vi "KB_GetCreatFlatnessXYZ.vi"(10 "Recent":dbl[](array[numeric]), 11 "Image Pixels (U8)":dbl[][](array[numeric])) -> (3 "Create Flatnesss Base Point":cluster{"X":dbl, "Y":dbl, "Z":dbl}[](array[cluster]))   [LabVIEW 2015]
panel:
  out "输出簇":cluster{"X":dbl, "Y":dbl, "Z":dbl}
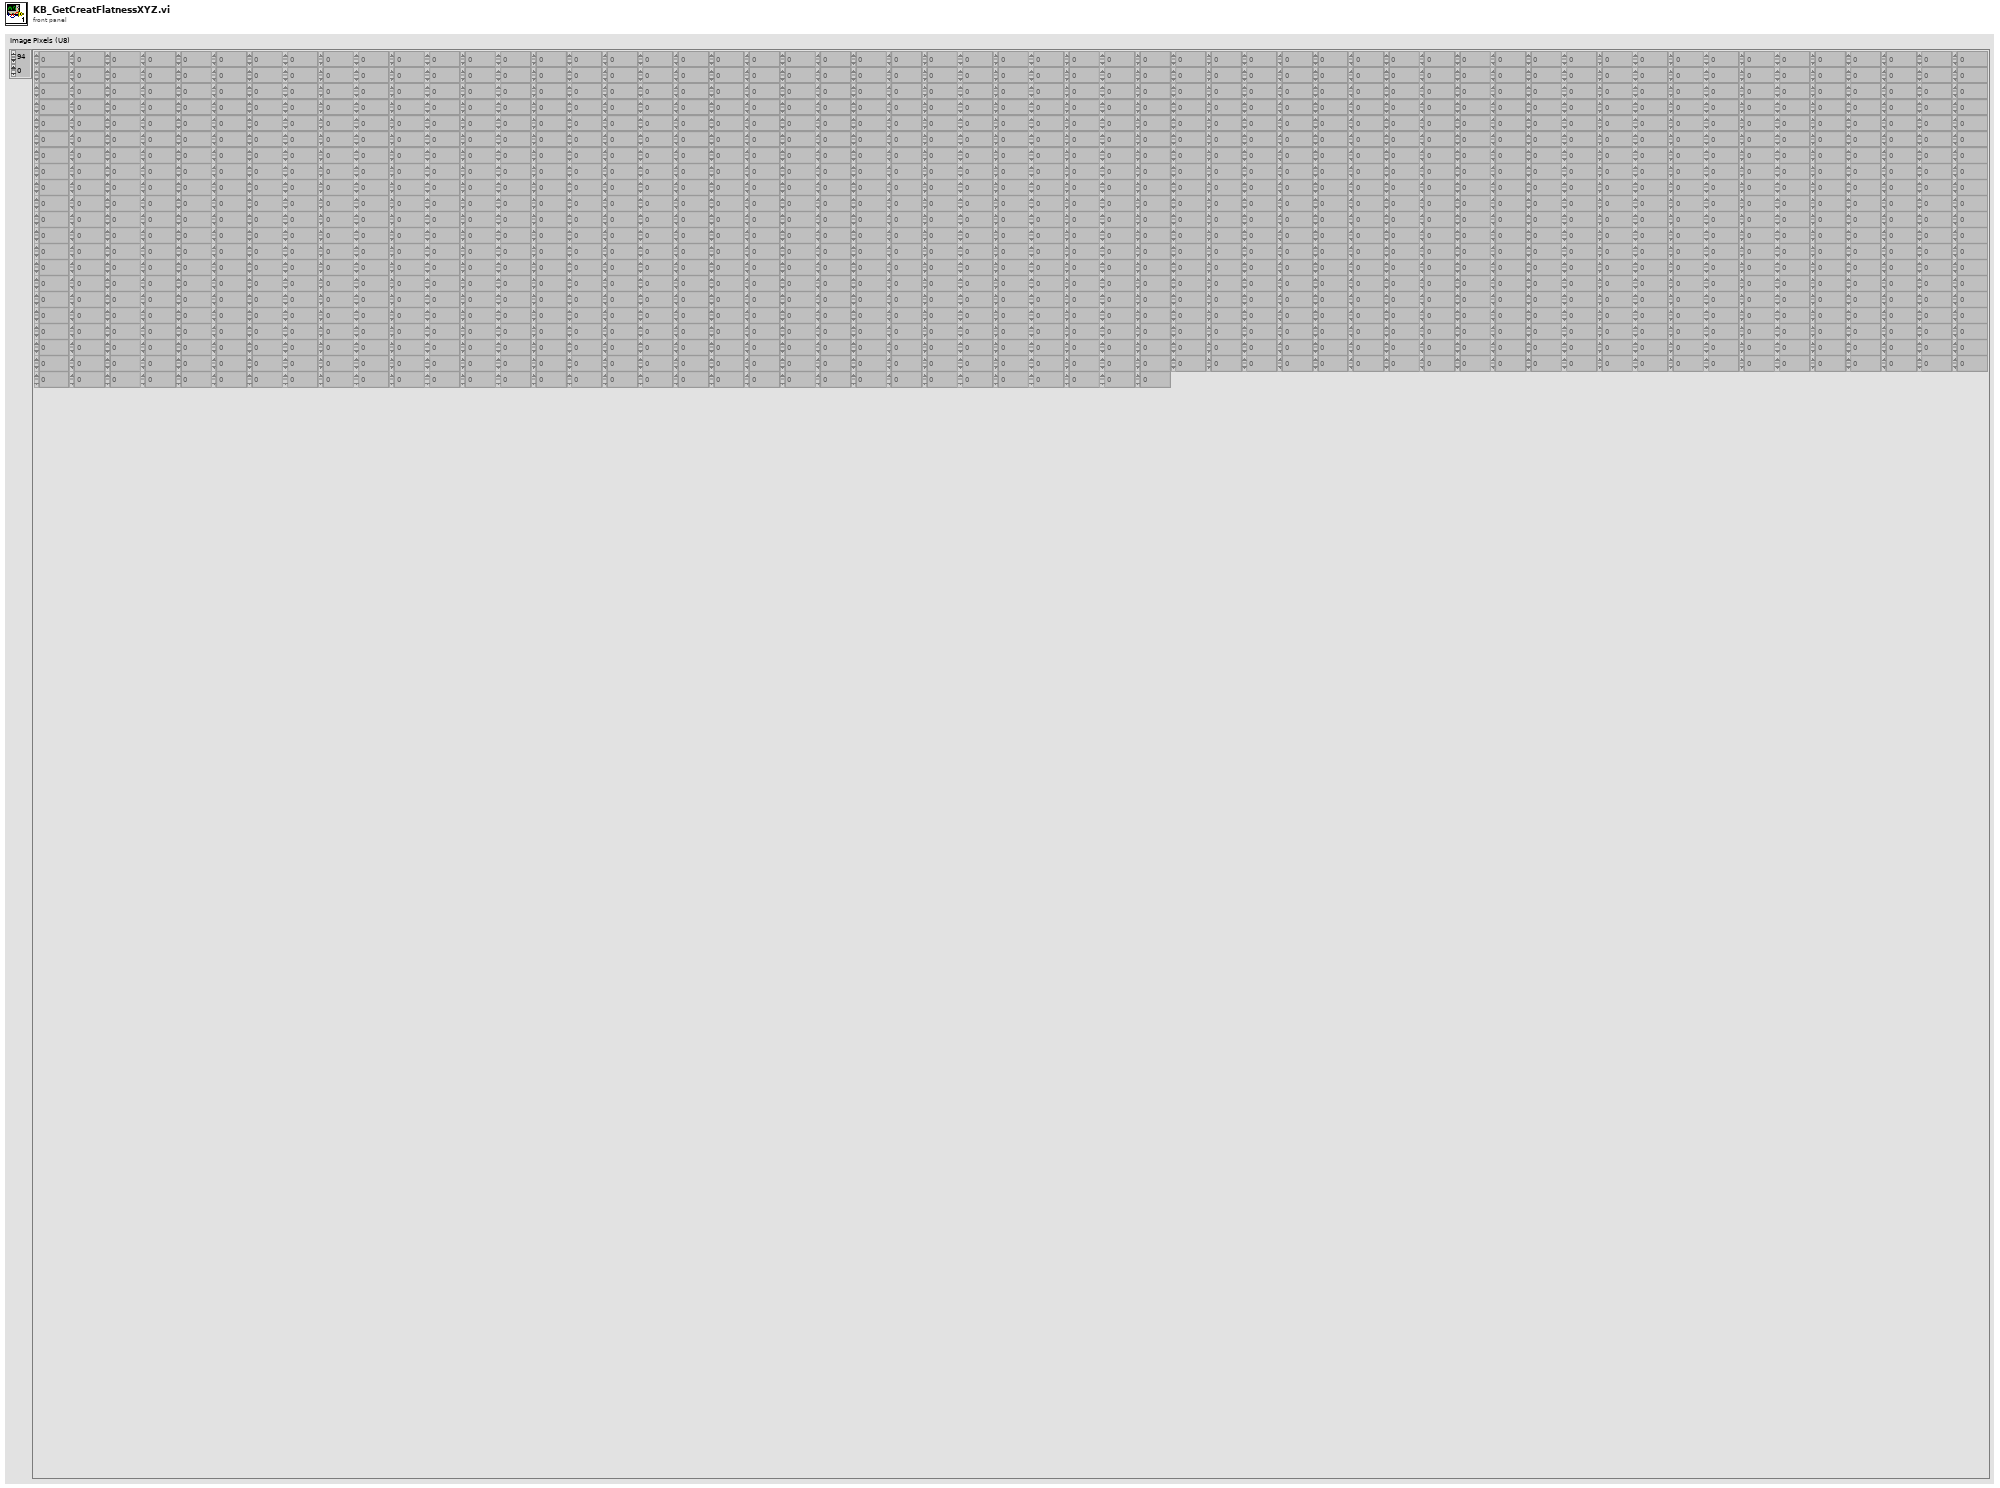
[diagram p1: front panel]
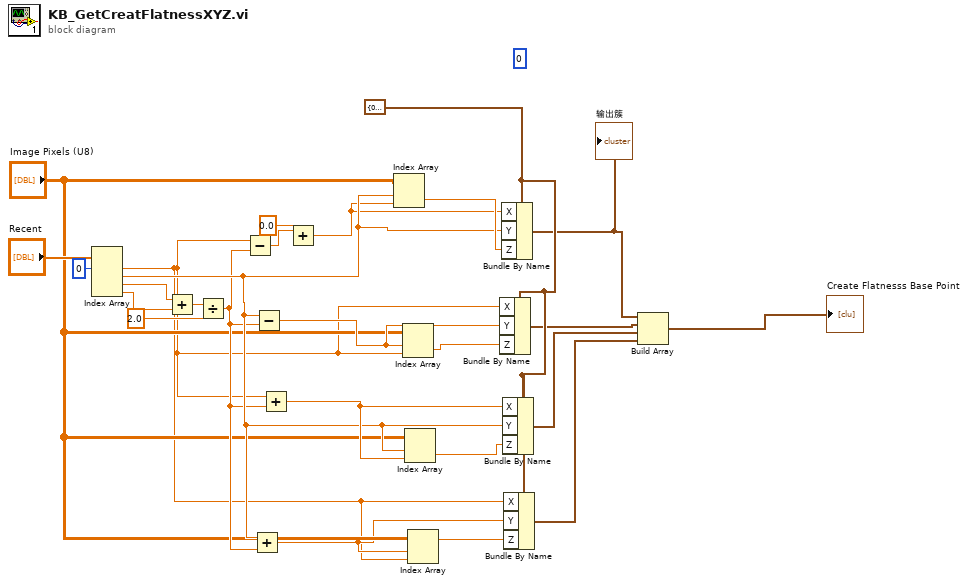
[diagram p0: block diagram]
diagram:
  (unwired) 0
  w15 = cluster{"X":dbl, "Y":dbl, "Z":dbl} {"X"=0.0, "Y"=0.0, "Z"=0.0}
  n1 = Index Array(array="Recent", index #1=0 ("索引")) -> (element #1=w10:dbl, element #2=w14:dbl, element #3=w24:dbl, element #4=w23:dbl)  [unwired: 3 in]
  n2 = Add(x=w24, y=w23) -> (x+y=w22:dbl)
  n3 = Divide(x=w22, y=2.0) -> (x/y=w13:dbl)
  n4 = Subtract(x=w10, y=w13) -> (x-y=w3:dbl)
  n5 = Add(x=w14, y=w13) -> (x+y=w11:dbl)
  n6 = Subtract(x=w14, y=w13) -> (x-y=w18:dbl)
  n7 = Add(x=w10, y=w13) -> (x+y=w17:dbl)
  n8 = Add(x=w3, y=0.0) -> (x+y=w1:dbl)
  n9 = Index Array(array="Image Pixels (U8)", index (row)=w14, index (col)=w1) -> (element=w20:dbl)
  n10 = Index Array(array="Image Pixels (U8)", index (row)=w18, index (col)=w10) -> (element=w19:dbl)
  n11 = Index Array(array="Image Pixels (U8)", index (row)=w14, index (col)=w17) -> (element=w16:dbl)
  n12 = Index Array(array="Image Pixels (U8)", index (row)=w11, index (col)=w10) -> (element=w5:dbl)
  n13 = Bundle By Name(cluster=w15, "X"=w10, "Y"=w18, "Z"=w19) -> (w8:cluster{"X":dbl, "Y":dbl, "Z":dbl})
  n14 = Bundle By Name(cluster=w15, "X"=w1, "Y"=w14, "Z"=w20) -> (w9:cluster{"X":dbl, "Y":dbl, "Z":dbl})
  "输出簇" <- w9
  n15 = Bundle By Name(cluster=w15, "X"=w17, "Y"=w14, "Z"=w16) -> (w7:cluster{"X":dbl, "Y":dbl, "Z":dbl})
  n16 = Bundle By Name(cluster=w15, "X"=w10, "Y"=w11, "Z"=w5) -> (w6:cluster{"X":dbl, "Y":dbl, "Z":dbl})
  n17 = Build Array(w9, w8, w7, w6) -> (→"Create Flatnesss Base Point":cluster{"X":dbl, "Y":dbl, "Z":dbl}[])
